vi "Write Show FP_.vi"(8 "error in (no error)":errorcluster, 10 "Show FP?":refnum<vi>, 11 "Measurement UI in":refnum<class "Measurement UI.lvclass">) -> (0 "error out":errorcluster, 3 "Measurement UI out":refnum<class "Measurement UI.lvclass">)   [LabVIEW 2017, in "Measurement UI.lvlib" / "Measurement UI.lvclass"]
uses:
  Measurement UI.lvclass
  Measurement UI.lvclass/Measurement UI.ctl
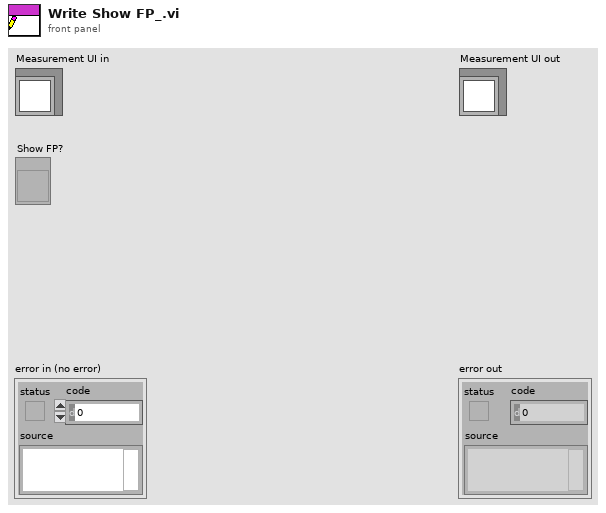
[diagram p1: front panel]
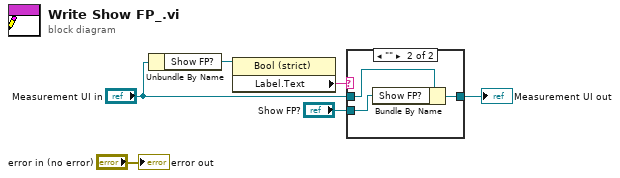
[diagram p0: block diagram]
diagram:
  n1 = Unbundle By Name("Measurement UI in") -> ("Show FP?"=w3:refnum<vi>)
  n2 = property class="Bool (strict)"(reference=w3) -> ("Label.Text"=w1:string)  [unwired: 1 in, 2 out]
  n3 = case shown="\"\"" w1 {
    tunnel: [w7 w9] -> w6
    tunnel: "Measurement UI in" -> [w7 w10]
    tunnel: "Show FP?" -> [_ w8]
    frame Default {
    }
    frame "" {
      n4 = Bundle By Name(cluster=w10, "Show FP?"=w8) -> (w9:refnum<class "Measurement UI.lvclass">)
    }
  }
  "Measurement UI out" <- w6
  "error out" <- "error in (no error)"
